vi "(SubVI)I2C_16Bit-8Bit_Write_Array.vi"(5 "Log Ref":refnum<vi>, 7 "Clock":T2=enum."400kHz", 8 "error in (no error)":errorcluster caption="에러 입력(에러 없음)", 9 "Data to Write":T1[](array[typedef]) {"Address" format="%04x"; "Data" format="%02x"}, 11 "ID":u8) -> (0 "error out":errorcluster caption="에러 출력", 2 "Log out":string)   [LabVIEW 2020]
uses:
  Controls/(Ctrl)I2C_Clock.ctl
  Controls/(Ctrl)I2C_16Bit-8Bit_Write Array.ctl
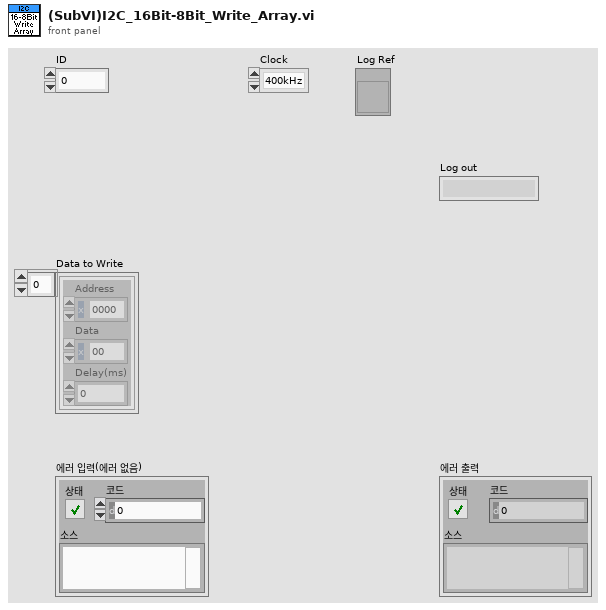
[diagram p1: front panel]
types:
  T1 = typedef "(Ctrl)I2C_16Bit-8Bit_Write Array.ctl" = cluster{"Address":u16, "Data":u8, "Delay(ms)":i32}
  T2 = typedef "(Ctrl)I2C_Clock.ctl" = enum8{"1MHz", "2MHz", "3MHz", "400kHz"}
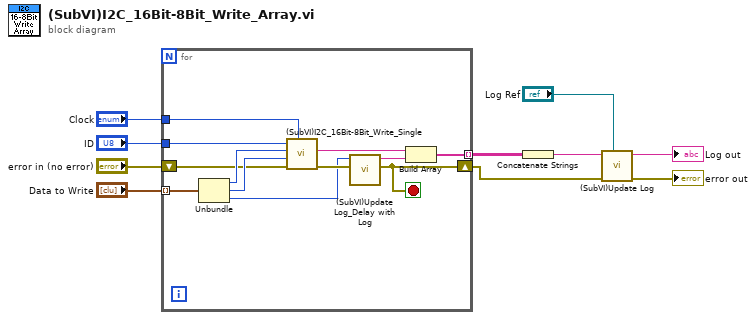
[diagram p0: block diagram]
diagram:
  n1 = for {
    tunnel: "Clock" -> [w22]
    tunnel: "ID" -> [w21]
    tunnel: "Data to Write" -> [w20] mode=indexing
    shift-right: [w14] -> w3
    shift-left: "error in (no error)" -> [w15]
    tunnel: [w12] -> w6 mode=indexing
    stop <- w14 stop-if-true
    n2 = Unbundle(w20) -> ("Address"=w19:u16, "Data"=w18:u8, "Delay(ms)"=w16:i32)
    n3 = call "(SubVI)I2C_16Bit-8Bit_Write_Single.vi"("Clock"=w22, "error in (no error)"=w15, "Data to Write"=w18, "Address"=w19, "ID"=w21) -> ("error out"=w17:errorcluster, "Log"=w13:string)  [unwired: 5 in]
    n4 = call "(SubVI)Update Log_Delay with Log.vi"("error in (no error)"=w17, "Delay (ms)"=w16) -> ("error out"=w14:errorcluster, "Log"=w11:string)  [unwired: 8 in]
    n5 = Build Array(w13, w11) -> (w12:string[])
  }
  n6 = Concatenate Strings(w6) -> (w5:string)
  n7 = call "(SubVI)Update Log.vi"("Log Ref"="Log Ref", "error in (no error)"=w3, "Log"=w5) -> ("error out"=→"error out":errorcluster, "Log out"=→"Log out":string)  [unwired: 7 in]
